vi "Read Single-Point.vi"(8 "error in (no error)":errorcluster, 10 "maximum time (5s)":dbl[unit]=5000.0 caption="maximum time (5000 ms)", 11 "CS++DMM in":refnum<class "CS++DMM.lvclass">) -> (0 "error out":errorcluster, 2 "reading":dbl format="%^.2e", 3 "CS++DMM out":refnum<class "CS++DMM.lvclass">)   [LabVIEW 2013, in "CS++DMM.lvlib" / "CS++DMM.lvclass"]
doc: "This VI initiates a measurement, waits until the DMM has returned to the Idle state, and returns the measured value.\n\nThis VI applies default values to properties that have not been set by the user under the following conditions:\n\n(1) If the user has not set the value of any property in the IviDmmMultiPoint extension group, the VI sets the IviDmm>>Multi-Point Acquisition>>Sample Count [MP] and IviDmm>>Multi-Point Acquisition>>Trigger Count [MP] properties to 1.\n\n(2) If the user has not set the value of the IviDmm>Measurement Operation Options>Auto Zero [AZ] property, the VI sets the value of this property to IVIDMM_VAL_AUTO_ZERO_OFF (0). \n\nNotes:\n\n(1) After this VI executes, the Reading parameter contains an actual reading or a value indicating that an over-range condition occurred.\n\n(2) If an over-range condition occurs, the Reading parameter contains an IEEE defined NaN (Not a Number) value and the VI returns the IVIDMM_WARN_OVER_RANGE (0x3ffA2001) warning code.\n\n(3) You can test the measurement value for an over-range condition by calling the IviDmm Is Over-Range VI.\n\n(4) This VI performs interchangeability checking when the IviDmm>>Inherent IVI Settings>>User Options>>Interchange Check property is set to TRUE. If the IviDmm>>Inherent IVI Settings>>User Options>>Spy property is set to TRUE, you use the NI Spy utility to view interchangeability warnings. You use the IviDmm Get Next Interchange Warning VI to retrieve interchangeability warnings when the IviDmm>>Inherent IVI Settings>>User Options>>Spy property is set to FALSE. For more information about interchangeability checking, refer to the help text for the IviDmm>>Inherent IVI Settings>>User Options>>Interchange Check property.\n\n(5) The class driver returns a simulated measurement when this VI is called and the IviDmm>>Inherent IVI Settings>>User Options>>Simulate property is set to TRUE and the IviDmm>>Inherent IVI Settings>>User Options>>Use Specific Simulation property is set to FALSE. For information on how to configure a simulated measurement, refer to the online help manual."
uses:
  CS++DMM.lvclass
  CS++DMM.lvclass/CS++DMM.ctl
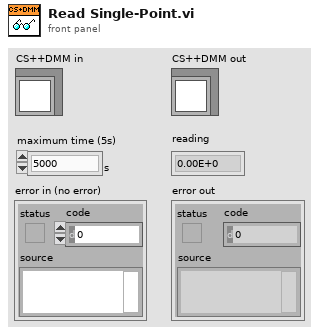
[diagram p1: front panel]
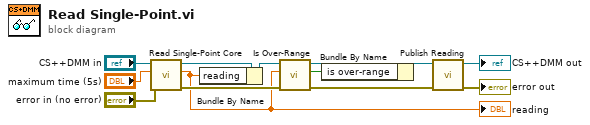
[diagram p0: block diagram]
diagram:
  n1 = call-dynamic "Read Single-Point Core.vi"("error in (no error)"="error in (no error)", "maximum time (5s)"="maximum time (5s)", "CS++DMM in"="CS++DMM in") -> ("error out"=w6:errorcluster, "reading"=w4:dbl, "CS++DMM out"=w8:refnum<class "CS++DMM.lvclass">)  [unwired: 6 in]
  "reading" <- w4
  n2 = Bundle By Name(cluster=w8, "reading"=w4) -> (w7:refnum<class "CS++DMM.lvclass">)
  n3 = call-dynamic "Is Over-Range.vi"("error in (no error)"=w6, "measurement value"=w4, "CS++DMM in"=w7) -> ("error out"=w5:errorcluster, "is over-range"=w1:bool, "CS++DMM out"=w3:refnum<class "CS++DMM.lvclass">)  [unwired: 6 in]
  n4 = Bundle By Name(cluster=w3, "is over-range"=w1) -> (w2:refnum<class "CS++DMM.lvclass">)
  n5 = call "Publish Reading.vi"("error in (no error)"=w5, "CS++DMM in"=w2) -> ("error out"=→"error out":errorcluster, "CS++DMM out"=→"CS++DMM out":refnum<class "CS++DMM.lvclass">)  [unwired: 8 in]
